vi "Asylum_Driver_GetImagingMode.vi"(8 "error in (no error)":errorcluster, 11 "Application In":refnum<k7>) -> (0 "error out":errorcluster, 2 "Imaging Mode":string, 3 "Application Out":refnum<k7>)   [LabVIEW 2019]
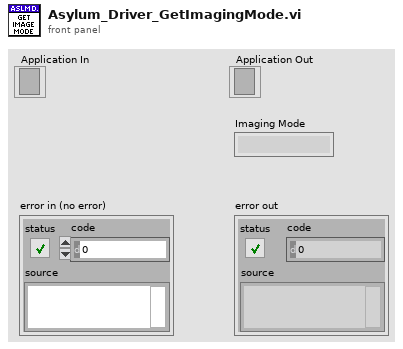
[diagram p1: front panel]
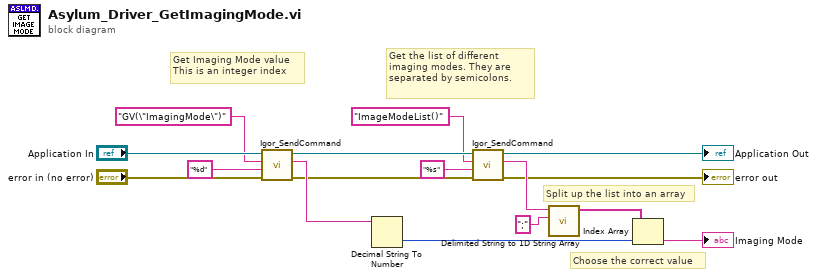
[diagram p0: block diagram]
diagram:
  # "Choose the correct value"
  # "Split up the list into an array"
  # "Get the list of different imaging modes. They are separated by semicolons."
  # "Get Imaging Mode value\nThis is an integer index"
  n1 = call <userlib>:"Igor_SendCommand.vi"("error in (no error)"="error in (no error)", "Format"="%d", "command"="GV(\"ImagingMode\")", "Application In"="Application In") -> ("error out"=w3:errorcluster, "results"=w12:string, "Application Out"=w9:refnum<k7>)  [unwired: 4 in, 1 out]
  n2 = Decimal String To Number(string=w12) -> (number=w11:i32)  [unwired: 2 in, 1 out]
  n3 = call <userlib>:"Igor_SendCommand.vi"("error in (no error)"=w3, "Format"="%s", "command"="ImageModeList()", "Application In"=w9) -> ("error out"=→"error out":errorcluster, "results"=w15:string, "Application Out"=→"Application Out":refnum<k7>)  [unwired: 4 in, 1 out]
  n4 = call <vilib>:"Delimited String to 1D String Array.vi"("delimiter"=";", "delimited string"=w15) -> ("string array"=w7:string[])  [unwired: 9 in]
  n5 = Index Array(array=w7, index=w11) -> (element=→"Imaging Mode":string)
